vi "Scan Export.vi"(7 "Which Data To Include (0: Format)":i32(ring) items=["Format", "Relative", "Raw", "Stamp", "All", "Standard", "Brief", "Extra", "Status", "Chancol", "Easygraph"], 8 "error in (no error)":errorcluster, 9 "When To Write  (0: Step)":i32(ring) items=["Step", "Scan", "End", "Never"], 10 "File Name (\"\")":string, 11 "VISA resource name":refnum<visa-resource-name>) -> (0 "error out":errorcluster, 3 "VISA resource name out":refnum<visa-resource-name>)   [LabVIEW 2020, in "Keithley DMM6500 DAQ6500 Series.lvlib"]
doc: "Starts a scan and dumps the data to a file on a thumb drive"
uses:
  <instrlib>/Keithley DMM6500 DAQ6500 Series/Keithley DMM6500 DAQ6500 Series.lvlib
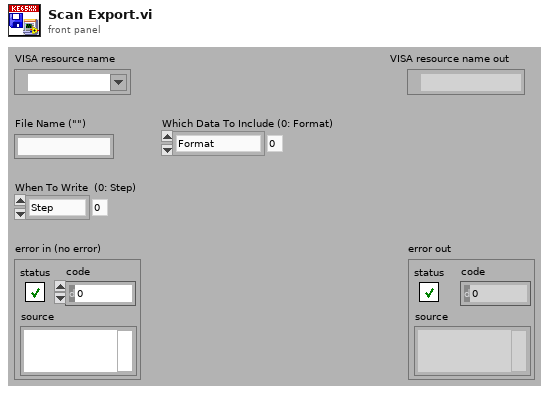
[diagram p1: front panel]
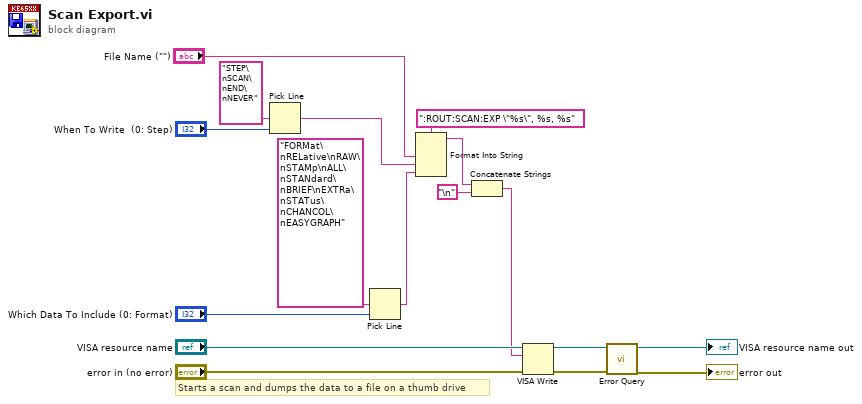
[diagram p0: block diagram]
diagram:
  # "Starts a scan and dumps the data to a file on a thumb drive"
  n1 = Pick Line(multi-line string="STEP\nSCAN\nEND\nNEVER", line index="When To Write  (0: Step)") -> (output string=w6:string)  [unwired: 1 in]
  n2 = Pick Line(multi-line string="FORMat\nRELative\nRAW\nSTAMp\nALL\nSTANdard\nBRIEF\nEXTRa\nSTATus\nCHANCOL\nEASYGRAPH", line index="Which Data To Include (0: Format)") -> (output string=w5:string)  [unwired: 1 in]
  n3 = Format Into String(format string=":ROUT:SCAN:EXP \"%s\", %s, %s", "File Name (\"\")", w6, w5) -> (resulting string=w8:string)  [unwired: 2 in, 1 out]
  n4 = Concatenate Strings(w8, "\n") -> (w9:string)
  n5 = VISA Write(VISA resource name="VISA resource name", write buffer=w9, error in (no error)="error in (no error)") -> (VISA resource name out=w13:refnum<visa-resource-name>, error out=w12:errorcluster)  [unwired: 1 out]
  n6 = call <instrlib>:"Error Query.vi"("error in (no error)"=w12, "VISA resource name"=w13) -> ("error out"=→"error out":errorcluster, "VISA resource name out"=→"VISA resource name out":refnum<visa-resource-name>)  [unwired: 6 in, 2 out]
